vi "Vibrometer_Thermocouple_firstVI.vi"() -> ()   [LabVIEW 2017]
panel:
  out "Thermo couple":dynamicdata(graph)
  in  "Displacement Scale (mm/V)":dbl
  out "Room Temp":dynamicdata(graph)
  out "Disp":dynamicdata(graph)
  in  "stop":bool
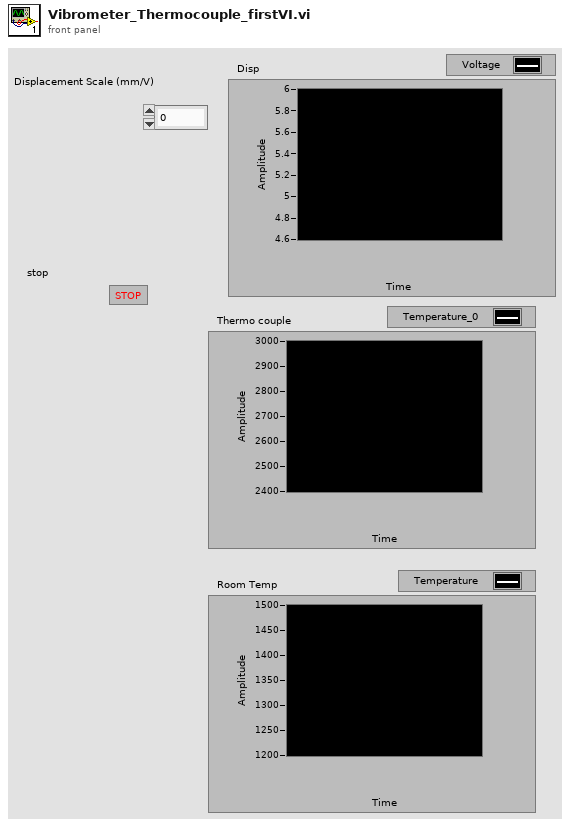
[diagram p1: front panel]
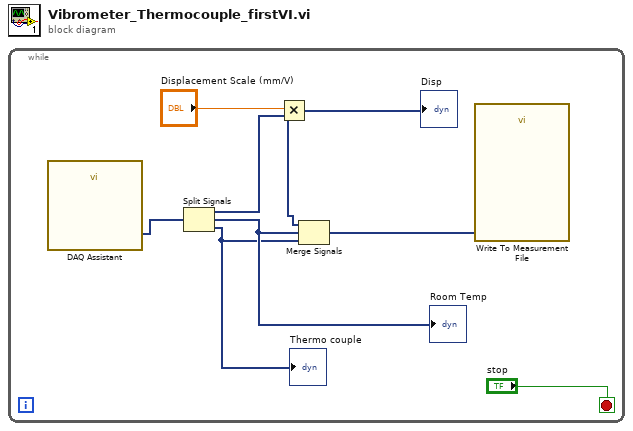
[diagram p0: block diagram]
diagram:
  n1 = while {
    stop <- "stop" stop-if-true
    n2 = call "DAQ Assistant"() -> ("data"=w7:dynamicdata)  [unwired: 17 in, 2 out]
    n3 = Split Signals(w7) -> (w5:dynamicdata, w4:dynamicdata, w3:dynamicdata)  [unwired: 3 in]
    "Room Temp" <- w4
    "Thermo couple" <- w3
    n4 = Multiply(x="Displacement Scale (mm/V)", y=w5) -> (x*y=w2:dynamicdata)
    "Disp" <- w2
    n5 = Merge Signals(w2, w4, w3) -> (w1:dynamicdata)
    n6 = call "Write To Measurement File"("Signals"=w1) -> ()  [unwired: 16 in, 3 out]
  }
